vi "NetVarWrite_str.vi"(8 "error in (no error)":errorcluster, 10 "String":string, 11 "Refnum in":refnum<k21>) -> (0 "error out":errorcluster)   [LabVIEW 2016]
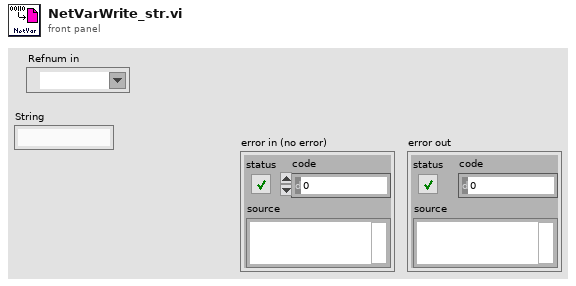
[diagram p1: front panel]
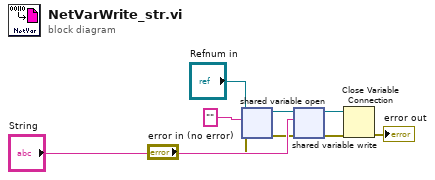
[diagram p0: block diagram]
diagram:
  n1 = shared-variable-open("Refnum in", "error in (no error)", "") -> (w5:refnum<k21>, w4:errorcluster)  [unwired: 1 in]
  n2 = shared-variable-write(w5, w4, "String") -> (w6:refnum<k21>, w3:errorcluster)
  n3 = Close Variable Connection(8:w3, 11:w6) -> (0:→"error out":errorcluster)
